vi "Write Both Fan States.vi"(8 "error in (no error)":cluster{"状态":bool, "代码":i32, "源":string} caption="错误输入（无错误）", 9 "风扇B状态":bool, 10 "风扇A状态":bool, 11 "硬件双风扇输入":refnum<class "HW Dual Fan.lvclass">) -> (0 "error out":cluster{"状态":bool, "代码":i32, "源":string} caption="错误输出")   [LabVIEW 2015, in "HW Dual Fan.lvclass"]
uses:
  HW Dual Fan.lvclass
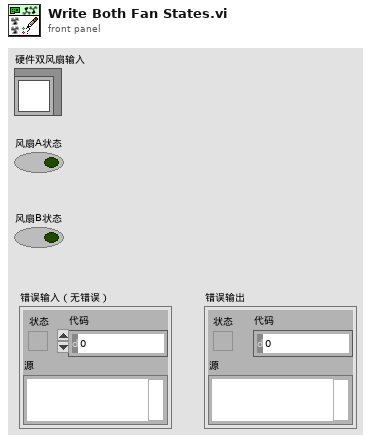
[diagram p1: front panel]
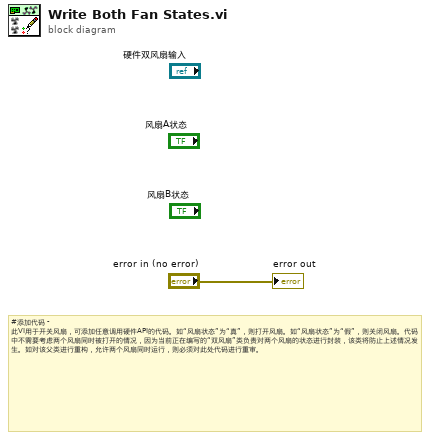
[diagram p0: block diagram]
diagram:
  # "#添加代码 - 此VI用于开关风扇，可添加任意调用硬件API的代码。如“风扇状态”为“真”，则打开风扇。如“风扇状态”为“假”，则关闭风扇。代码中不需要考虑两个风扇同时被打开的情况，因为当前正在编写的“双风扇”类负责对两个风扇的状态进行封装，该类将防止上述情况发生。如对该父类进行重构，允许两个风扇同时运行，则必须对此处代码进行重审。"
  "error out" <- "error in (no error)"
